vi "dataToBooleanArray.vi"(1 "Data":u8[](array[numeric])) -> (0 "Boolean array":bool[](array[boolean]))   [LabVIEW 2024, in "canopen.lvlib"]
doc: "Converts an arbitrary chunk of binary data to its boolean representation."
uses:
  canopen.lvlib
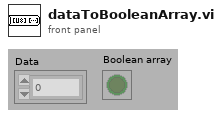
[diagram p1: front panel]
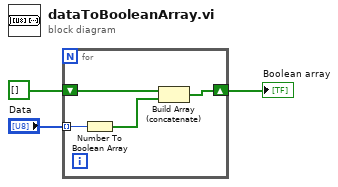
[diagram p0: block diagram]
diagram:
  n1 = for {
    tunnel: "Data" -> [w7] mode=indexing
    shift-right: [w4] -> w1
    shift-left: bool[] [] ("array") -> [w5]
    n2 = Number To Boolean Array(number=w7) -> (Boolean array=w6:bool[])
    n3 = Build Array (concatenate)(w5, w6) -> (w4:bool[])
  }
  "Boolean array" <- w1
